vi "NIDCPower_channel_ganging - output enabled.vi"(8 "error in (no error)":errorcluster, 9 "output enabled":bool=TRUE, 11 "Ganged Session In":T1) -> (0 "error out":errorcluster, 3 "Ganged Session Out":T1)   [LabVIEW 2021]
uses:
  ctl/NIDCPower_channel_ganging - ctl - ganged session.ctl
  ctl/NIDCPower_channel_ganging - ctl - ganged config.ctl
  ctl/NIDCPower_channel_ganging - ctl - channel mode.ctl
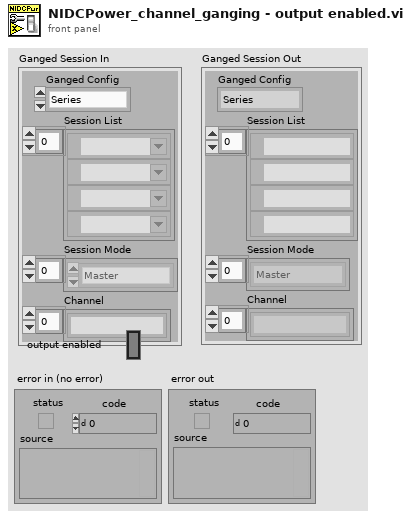
[diagram p1: front panel]
types:
  T1 = typedef "NIDCPower_channel_ganging - ctl - ganged session.ctl" = cluster{"Ganged Config":T2, "Session List":refnum<k15>[], "Session Mode":T3[], "Channel":string[]}
  T2 = typedef "NIDCPower_channel_ganging - ctl - ganged config.ctl" = enum32{"Series", "Parallel", "Manual"}
  T3 = typedef "NIDCPower_channel_ganging - ctl - channel mode.ctl" = enum32{"Master", "Slave", "Slave - Inverted"}
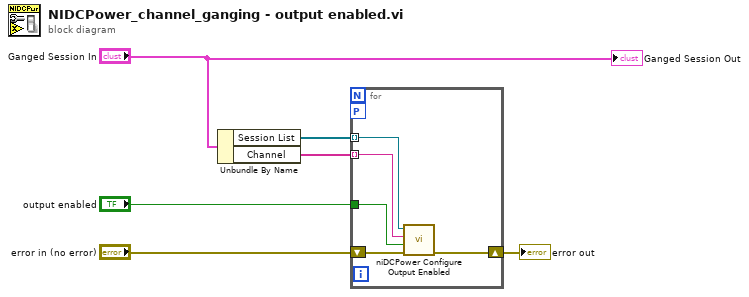
[diagram p0: block diagram]
diagram:
  n1 = Unbundle By Name("Ganged Session In") -> ("Session List"=w2:refnum<k15>[], "Channel"=w1:string[])
  n2 = for {
    shift-right: [w7] -> w5
    shift-left: "error in (no error)" -> [w11]
    tunnel: w2 -> [w10] mode=indexing
    tunnel: "output enabled" -> [w9]
    tunnel: w1 -> [w8] mode=indexing
    workers-P: _ -> [_]
    n3 = call <instrlib>:"niDCPower Configure Output Enabled.vi"("error in (no error)"=w11, "output enabled"=w9, "channel name"=w8, "instrument handle"=w10) -> ("error out"=w7:errorcluster)  [unwired: 6 in, 1 out]
  }
  "error out" <- w5
  "Ganged Session Out" <- "Ganged Session In"
